vi "DownsampleStage4_5782_10MHzPID.vi"(6 "Count to skip":u32=22, 8 "valid in":bool, 9 "reset":bool, 11 "Data in":fxp<+/-,32,14>[](array[numeric])=[0.0, 0.0, 0.0, 0.0, 0.0, 0.0]) -> (0 "valid out":bool, 3 "data out":fxp<+/-,32,14>[](array[numeric]))   [LabVIEW 2018]
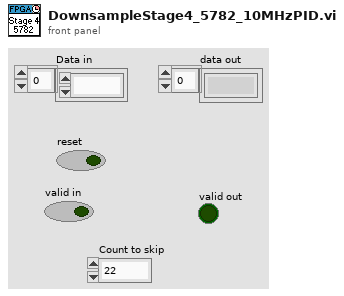
[diagram p1: front panel]
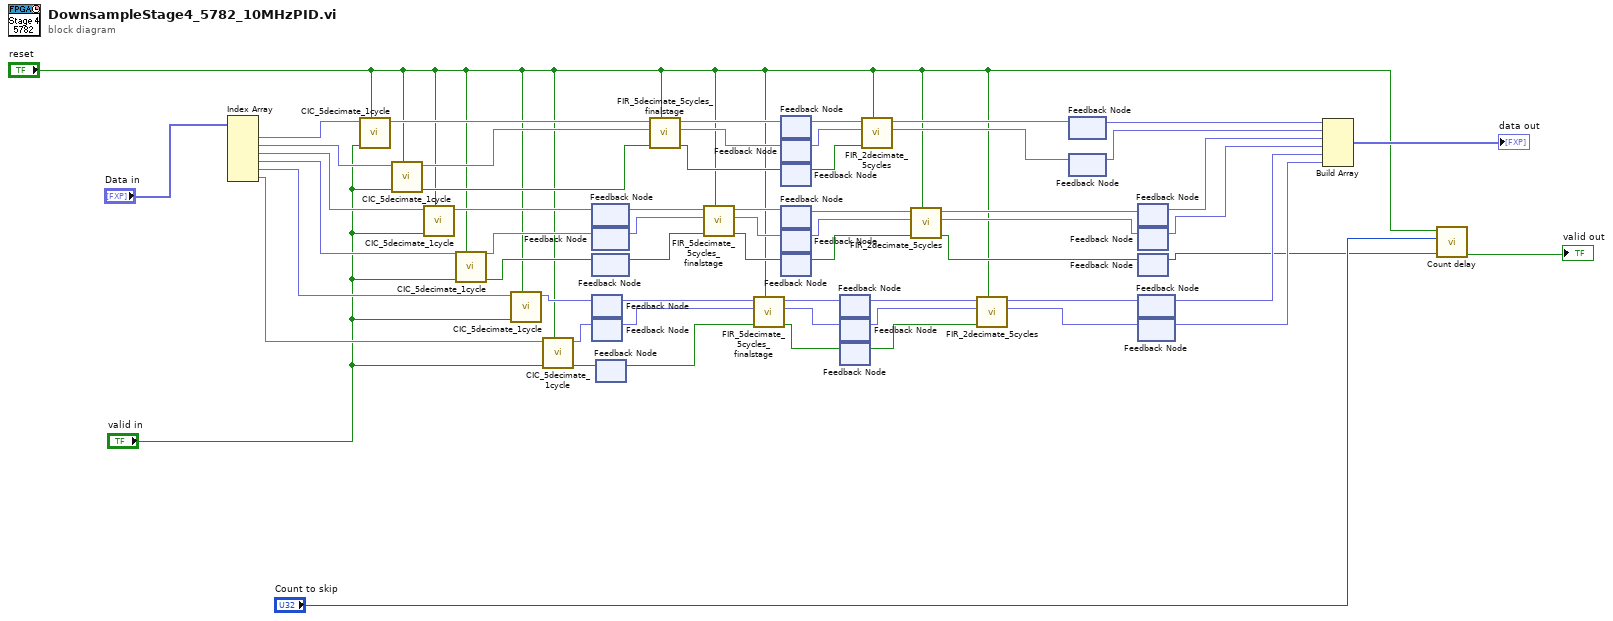
[diagram p0: block diagram]
diagram:
  n1 = Index Array(array="Data in") -> (element #1=w58:fxp<+/-,32,14>, element #2=w56:fxp<+/-,32,14>, element #3=w55:fxp<+/-,32,14>, element #4=w54:fxp<+/-,32,14>, element #5=w40:fxp<+/-,32,14>, element #6=w39:fxp<+/-,32,14>)  [unwired: 6 in]
  n2 = call "CIC_5decimate_1cycle.vi"("reset"="reset", "valid in"="valid in", "Data in"=w58) -> ("Data out"=w47:fxp<+/-,32,14>)  [unwired: 7 in, 1 out]
  n3 = call "CIC_5decimate_1cycle.vi"("reset"="reset", "valid in"="valid in", "Data in"=w56) -> ("valid out"=w45:bool, "Data out"=w46:fxp<+/-,32,14>)  [unwired: 7 in]
  n4 = call "CIC_5decimate_1cycle.vi"("reset"="reset", "valid in"="valid in", "Data in"=w55) -> ("Data out"=w53:fxp<+/-,32,14>)  [unwired: 7 in, 1 out]
  n5 = call "CIC_5decimate_1cycle.vi"("reset"="reset", "valid in"="valid in", "Data in"=w54) -> ("valid out"=w51:bool, "Data out"=w52:fxp<+/-,32,14>)  [unwired: 7 in]
  n6 = call "CIC_5decimate_1cycle.vi"("reset"="reset", "valid in"="valid in", "Data in"=w40) -> ("Data out"=w36:fxp<+/-,32,14>)  [unwired: 7 in, 1 out]
  n7 = call "CIC_5decimate_1cycle.vi"("reset"="reset", "valid in"="valid in", "Data in"=w39) -> ("valid out"=w32:bool, "Data out"=w35:fxp<+/-,32,14>)  [unwired: 7 in]
  n8 = feedback #1() -> (w50:fxp<+/-,32,14>)  [unwired: 1 in]
  n9 = feedback-in #1(w53) -> ()
  n10 = feedback #2() -> (w49:fxp<+/-,32,14>)  [unwired: 1 in]
  n11 = feedback-in #2(w52) -> ()
  n12 = feedback #3() -> (w48:bool)  [unwired: 1 in]
  n13 = feedback-in #3(w51) -> ()
  n14 = feedback #4() -> (w37:fxp<+/-,32,14>)  [unwired: 1 in]
  n15 = feedback-in #4(w36) -> ()
  n16 = feedback #5() -> (w38:fxp<+/-,32,14>)  [unwired: 1 in]
  n17 = feedback-in #5(w35) -> ()
  n18 = feedback #6() -> (w31:bool)  [unwired: 1 in]
  n19 = feedback-in #6(w32) -> ()
  n20 = call "FIR_5decimate_5cycles_finalstage.vi"("reset"="reset", "valid in"=w45, "Q in"=w46, "I in"=w47) -> ("valid out"=w21:bool, "Q out"=w22:fxp<+/-,32,14>, "I out"=w23:fxp<+/-,32,14>)  [unwired: 4 in, 1 out]
  n21 = call "FIR_5decimate_5cycles_finalstage.vi"("reset"="reset", "valid in"=w48, "Q in"=w49, "I in"=w50) -> ("valid out"=w13:bool, "Q out"=w14:fxp<+/-,32,14>, "I out"=w15:fxp<+/-,32,14>)  [unwired: 4 in, 1 out]
  n22 = call "FIR_5decimate_5cycles_finalstage.vi"("reset"="reset", "valid in"=w31, "Q in"=w38, "I in"=w37) -> ("valid out"=w4:bool, "Q out"=w5:fxp<+/-,32,14>, "I out"=w6:fxp<+/-,32,14>)  [unwired: 4 in, 1 out]
  n23 = feedback #7() -> (w26:fxp<+/-,32,14>)  [unwired: 1 in]
  n24 = feedback-in #7(w23) -> ()
  n25 = feedback #8() -> (w25:fxp<+/-,32,14>)  [unwired: 1 in]
  n26 = feedback-in #8(w22) -> ()
  n27 = feedback #9() -> (w24:bool)  [unwired: 1 in]
  n28 = feedback-in #9(w21) -> ()
  n29 = feedback #10() -> (w16:fxp<+/-,32,14>)  [unwired: 1 in]
  n30 = feedback-in #10(w15) -> ()
  n31 = feedback #11() -> (w17:fxp<+/-,32,14>)  [unwired: 1 in]
  n32 = feedback-in #11(w14) -> ()
  n33 = feedback #12() -> (w18:bool)  [unwired: 1 in]
  n34 = feedback-in #12(w13) -> ()
  n35 = feedback #13() -> (w9:fxp<+/-,32,14>)  [unwired: 1 in]
  n36 = feedback-in #13(w6) -> ()
  n37 = feedback #14() -> (w8:fxp<+/-,32,14>)  [unwired: 1 in]
  n38 = feedback-in #14(w5) -> ()
  n39 = feedback #15() -> (w7:bool)  [unwired: 1 in]
  n40 = feedback-in #15(w4) -> ()
  n41 = call "FIR_2decimate_5cycles.vi"("reset"="reset", "valid in"=w24, "Q in"=w25, "I in"=w26) -> ("Q out"=w19:fxp<+/-,32,14>, "I out"=w20:fxp<+/-,32,14>)  [unwired: 4 in, 2 out]
  n42 = call "FIR_2decimate_5cycles.vi"("reset"="reset", "valid in"=w18, "Q in"=w17, "I in"=w16) -> ("valid out"=w10:bool, "Q out"=w11:fxp<+/-,32,14>, "I out"=w12:fxp<+/-,32,14>)  [unwired: 4 in, 1 out]
  n43 = call "FIR_2decimate_5cycles.vi"("reset"="reset", "valid in"=w7, "Q in"=w8, "I in"=w9) -> ("Q out"=w2:fxp<+/-,32,14>, "I out"=w3:fxp<+/-,32,14>)  [unwired: 4 in, 2 out]
  n44 = feedback #16() -> (w44:fxp<+/-,32,14>)  [unwired: 1 in]
  n45 = feedback-in #16(w20) -> ()
  n46 = feedback #17() -> (w43:fxp<+/-,32,14>)  [unwired: 1 in]
  n47 = feedback-in #17(w19) -> ()
  n48 = feedback #18() -> (w41:fxp<+/-,32,14>)  [unwired: 1 in]
  n49 = feedback-in #18(w12) -> ()
  n50 = feedback #19() -> (w42:fxp<+/-,32,14>)  [unwired: 1 in]
  n51 = feedback-in #19(w11) -> ()
  n52 = feedback #20() -> (w28:bool)  [unwired: 1 in]
  n53 = feedback-in #20(w10) -> ()
  n54 = feedback #21() -> (w34:fxp<+/-,32,14>)  [unwired: 1 in]
  n55 = feedback-in #21(w3) -> ()
  n56 = feedback #22() -> (w33:fxp<+/-,32,14>)  [unwired: 1 in]
  n57 = feedback-in #22(w2) -> ()
  n58 = Build Array(w44, w43, w41, w42, w34, w33) -> (→"data out":fxp<+/-,32,14>[])
  n59 = call "Count delay.vi"("input valid"=w28, "Count to skip"="Count to skip", "Reset"="reset") -> ("output valid"=→"valid out":bool)  [unwired: 7 in, 1 out]
